vi "FPGA_display_QPD_signal.vi"(4 "QPD":T1, 5 "Reset":bool, 6 "error in":errorcluster) -> (0 "error out":errorcluster)   [LabVIEW 2015]
panel:
  out "Waveform Chart":cluster{"X":sgl, "Y":sgl, "SUM":sgl}(graph)
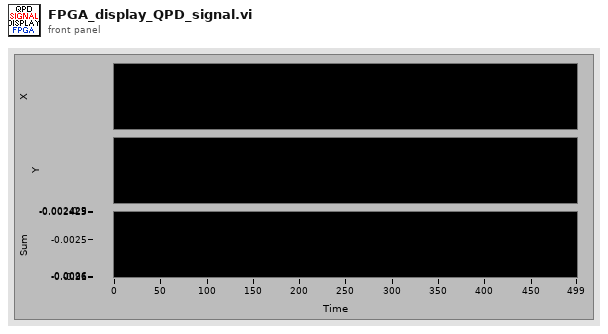
[diagram p1: front panel]
types:
  T1 = cluster{"X":sgl, "Y":sgl, "SUM":sgl, "count":u32}
  T2 = enum16{"Always On", "Always Off", "Off While Running"}
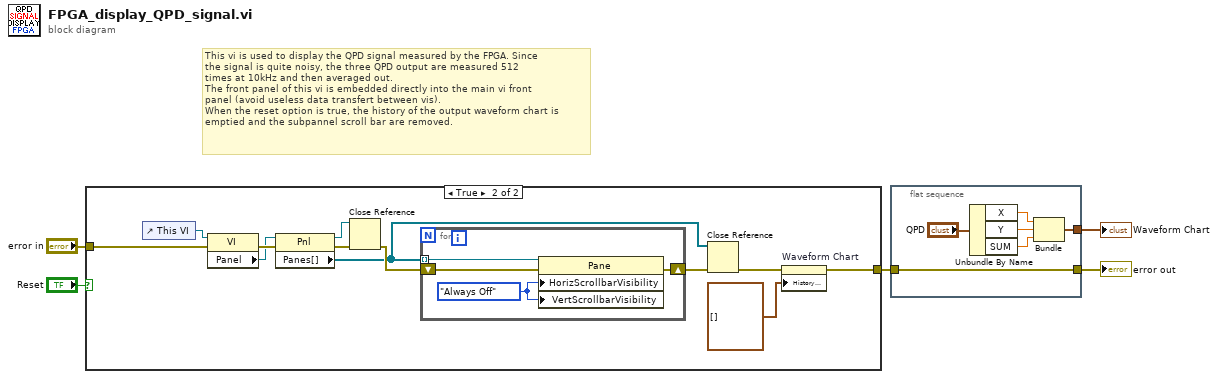
[diagram p0: block diagram]
diagram:
  # "This vi is used to display the QPD signal measured by the FPGA. Since\nthe signal is quite noisy, the three QPD output are measured 512\ntimes at 10kHz and then averaged out.\nThe front panel of this vi is embedded directly into the main vi front\npanel (avoid useless data transfert between vis). \nWhen the reset option is true, the history of the output waveform chart is\nemptied and the subpannel scroll bar are removed."
  n1 = case shown="True" "Reset" {
    tunnel: "error in" -> [w6 w10]
    tunnel: [w6 w7] -> w1
    frame False {
    }
    frame True {
      n2 = control-ref of="This VI"() -> (w11:refnum<vi>)
      n3 = property class="VI"(reference=w11, error in=w10) -> (error out=w13:errorcluster, "Panel"=w12:refnum<vi>)  [unwired: 1 out]
      n4 = property class="Pnl"(reference=w12, error in=w13) -> (reference out=w14:refnum<vi>, error out=w15:errorcluster, "Panes[]"=w17:refnum<vi>[])
      n5 = Close Reference(reference=w14, error in (no error)=w15) -> (error out=w18:errorcluster)
      n6 = for {
        tunnel: w17 -> [w22] mode=indexing
        shift-right: [w20] -> w16
        shift-left: w18 -> [w19]
        w21 = T2."Always Off" ("Horizontal Scrollbar Visibility")
        n7 = property class="Pane"(reference=w22, error in=w19, "HorizScrollbarVisibility"=w21, "VertScrollbarVisibility"=w21) -> (error out=w20:errorcluster)  [unwired: 1 out]
      }
      n8 = Close Reference(reference=w17, error in (no error)=w16) -> (error out=w9:errorcluster)
      n9 = property on="Waveform Chart" class="WFChart (strict)"(error in=w9, "History Data"=cluster{"mean":dbl, "mean":dbl, "mean":dbl}[] []) -> (error out=w7:errorcluster)  [unwired: 1 in, 1 out]
    }
  }
  n10 = flat-sequence {
    tunnel: [w28] -> w3
    tunnel: w1 -> [w28]
    tunnel: [w23] -> w2
    frame #0 {
      n11 = Unbundle By Name("QPD") -> ("X"=w25:sgl, "Y"=w26:sgl, "SUM"=w24:sgl)
      n12 = Bundle("X"=w25, "Y"=w26, "SUM"=w24) -> (w23:cluster{"X":sgl, "Y":sgl, "SUM":sgl})  [unwired: 1 in]
    }
  }
  "Waveform Chart" <- w2
  "error out" <- w3
